vi "NegJKflipFlop.vi"(6 "R":bool, 7 "S":bool, 9 "K":bool, 10 "Clk":bool, 11 "J":bool) -> (2 "Q":bool, 3 "/Q\\":bool)   [LabVIEW 2012]
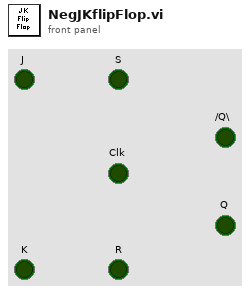
[diagram p1: front panel]
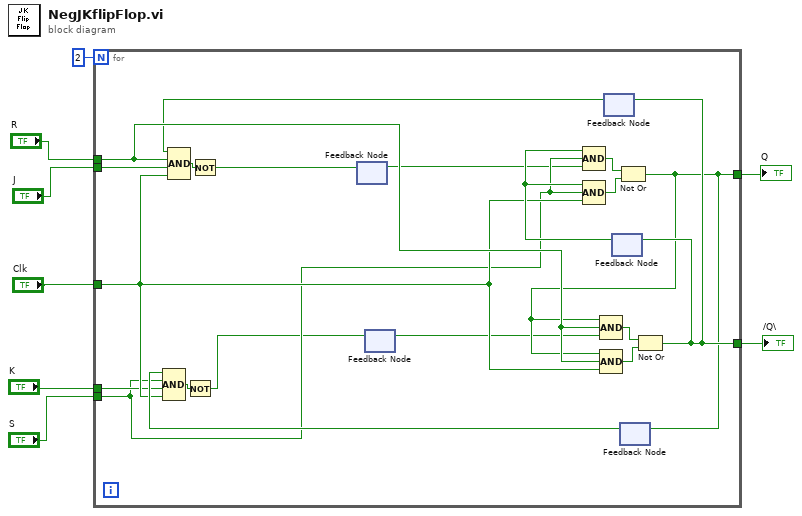
[diagram p0: block diagram]
diagram:
  n1 = for {
    N: 2 -> [_]
    tunnel: "J" -> [w28]
    tunnel: "K" -> [w16]
    tunnel: "Clk" -> [w17]
    tunnel: "R" -> [w21]
    tunnel: "S" -> [w15]
    tunnel: [w14] -> w3
    tunnel: [w13] -> w2
    n2 = feedback #1() -> (w9:bool)  [unwired: 1 in]
    n3 = feedback #2() -> (w12:bool)  [unwired: 1 in]
    n4 = feedback #3() -> (w19:bool)  [unwired: 1 in]
    n5 = Compound Arithmetic op=AND(w19, w21, w28, w17) -> (w27:bool)
    n6 = Not(x=w27) -> (.not. x?=w10:bool)
    n7 = feedback-in #1(w10) -> ()
    n8 = feedback #4() -> (w20:bool)  [unwired: 1 in]
    n9 = Compound Arithmetic op=AND(w20, w15, w9) -> (w25:bool)
    n10 = Compound Arithmetic op=AND(w20, w15, w17) -> (w24:bool)
    n11 = Not Or(1:w24, 2:w25) -> (0:w13:bool)
    n12 = Compound Arithmetic op=AND(w13, w21, w12) -> (w22:bool)
    n13 = Compound Arithmetic op=AND(w13, w21, w17) -> (w23:bool)
    n14 = feedback #5() -> (w18:bool)  [unwired: 1 in]
    n15 = Compound Arithmetic op=AND(w18, w15, w16, w17) -> (w26:bool)
    n16 = Not(x=w26) -> (.not. x?=w11:bool)
    n17 = feedback-in #2(w11) -> ()
    n18 = feedback-in #5(w13) -> ()
    n19 = Not Or(1:w23, 2:w22) -> (0:w14:bool)
    n20 = feedback-in #3(w14) -> ()
    n21 = feedback-in #4(w14) -> ()
  }
  "Q" <- w2
  "/Q\\" <- w3
